vi "指数电压信号.vi"() -> ()   [LabVIEW 2020]
doc: "I. Description:\nThis example demonstrates how to output multiple Voltage Updates (Samples) to an Analog Output Channel in a software timed loop.\n\nII. Instructions for Running:\n1. Select the Physical Channel to correspond to where your signal is output on the DAQ device.\n2. Enter the Minimum and Maximum Voltage Ranges\nNote: Use the Cont Acq Multiple Samples example to verify you are generating the correct output on the DAQ device.\n3. Set the loop rate.\n4. Run theVI.\n5. Stop the VI when desired.\n\nIII. Block Diagram Steps:\n1. Create an Analog Output Voltage channel.\n2. The Array Data is a sinewave with 1000 points, generates 5 cycles, and has an amplitude of 2.\n3. Call the Start VI\n4. Write one data point from the array (modulo indexed to loop count) until the user hits the stop button or an error occurs. The loop rate is settable to 1 millisecond. \n5. Call the Clear Task VI to clear the Task.\n6. Use the popup dialog box to display an error if any. \n\nIV. I/O Connections Overview:\nMake sure your signal output terminal matches the Physical Channel I/O Control. For further connection information, refer to your hardware reference manual."
uses:
  <vilib>/Analysis/polynomials.llb/Scalar Polynomial Evaluation (DBL).vi
  GlobalVariable.vi
  <vilib>/Analysis/NI_AALPro.lvlib
panel:
  in  "定值电压输出":bool
  in  "当前输出电压":dbl format="%#.4f"
  in  "倍周期(秒)":dbl=80.0
  in  "开始":bool
  in  "输出通道选择":u16(ring) items=["电压输出一", "电压输出二", "电压输出三", "电压输出四"]
  in  "V(0)电压(V)":dbl=0.1
  in  "Stop":bool caption="stop"
  in  "Loop Time (ms)":u32=200 caption="点间步长(mS)"
  out "XY Graph":cluster{"Y":dbl[], "Y":dbl[]}[](graph) caption="指数电压输出"
  # "V(t)=V(0)exp(t/Te)"
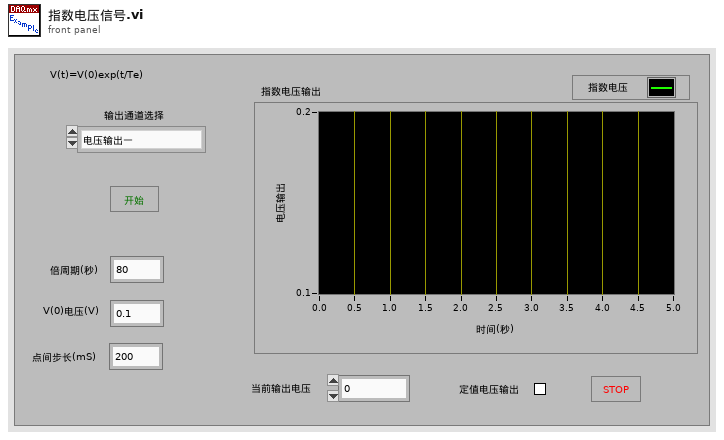
[diagram p1: front panel]
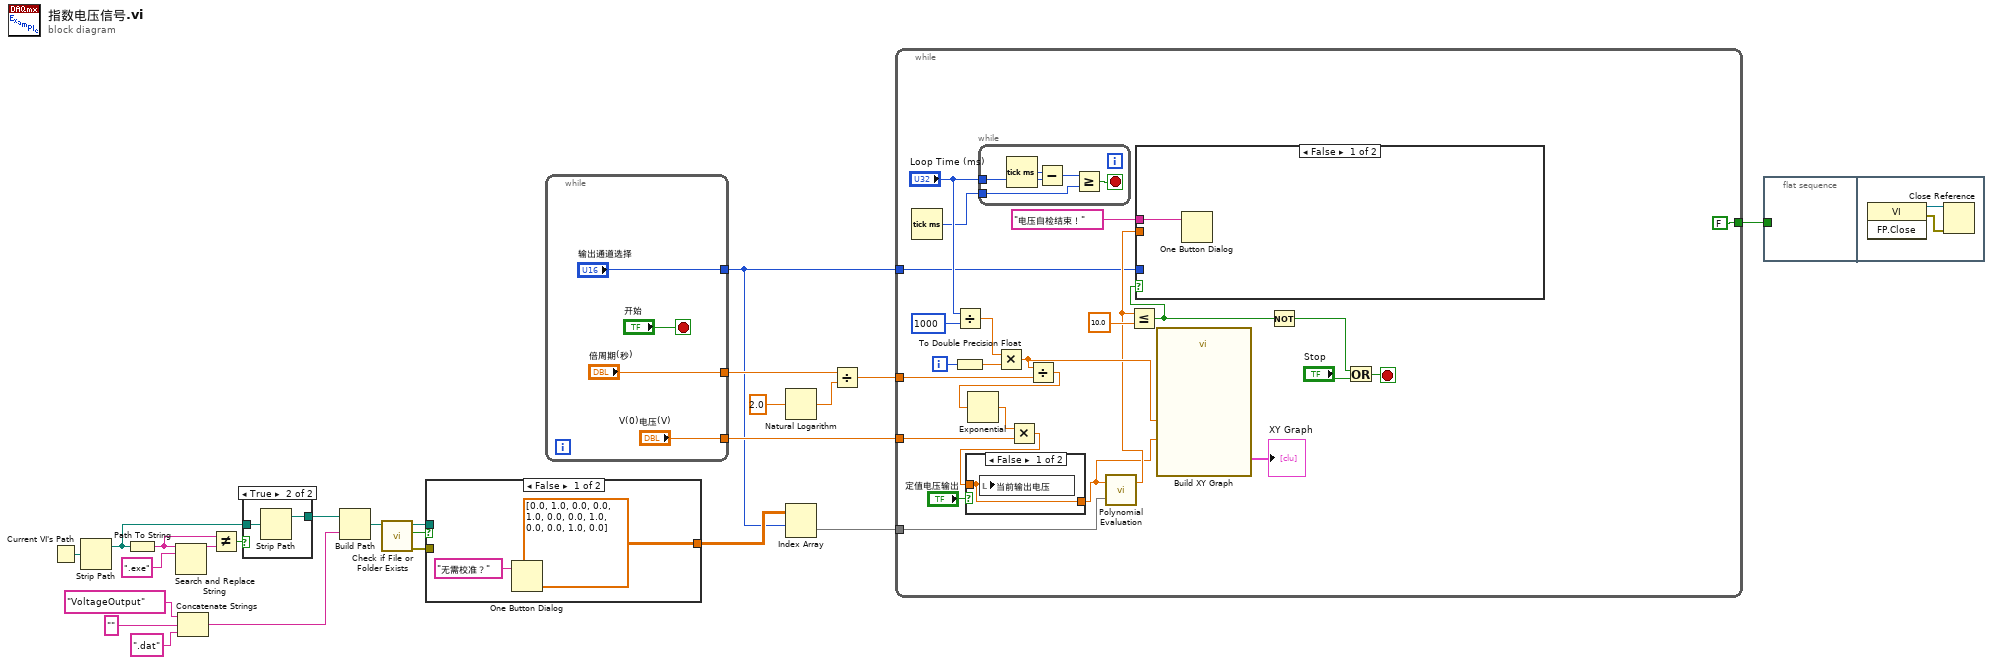
[diagram p0: block diagram]
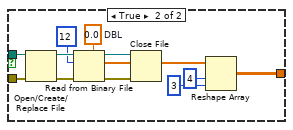
[diagram p2: hidden frame]
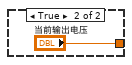
[diagram p4: hidden frame]
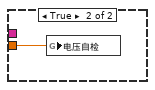
[diagram p5: hidden frame]
diagram:
  n1 = Current VI's Path() -> (path=w18:path)
  n2 = Strip Path(path=w18) -> (stripped path=w13:path)  [unwired: 1 out]
  n3 = Path To String(path=w13) -> (string=w15:string)
  n4 = Search and Replace String(input string=w15, search string=".exe" ("搜索字符串")) -> (result string=w16:string)  [unwired: 6 in, 3 out]
  n5 = Concatenate Strings("VoltageOutput", "" ("字符串"), ".dat") -> (w8:string)
  n6 = Not Equal?(x=w15, y=w16) -> (x != y?=w14:bool)
  n7 = case shown="True" w14 {
    tunnel: w13 -> [w25 w27]
    tunnel: [w25 w26] -> w12
    frame False {
    }
    frame True {
      n8 = Strip Path(path=w27) -> (stripped path=w26:path)  [unwired: 1 out]
    }
  }
  n9 = Build Path(base path=w12, name or relative path=w8) -> (appended path=w7:path)
  n10 = call <vilib>:"Check if File or Folder Exists.vi"("path"=w7) -> ("error out"=w5:errorcluster, "file or folder exists?"=w4:bool, "dup path"=w6:path)  [unwired: 8 in]
  n11 = case shown="False" w4 {
    tunnel: [dbl[][] [[0.0, 1.0, 0.0], [0.0, 1.0, 0.0], [0.0, 1.0, 0.0], [0.0, 1.0, 0.0]] w34] -> w11
    tunnel: w6 -> [_ w31]
    tunnel: w5 -> [_ w30]
    frame False {
      n12 = One Button Dialog(message="无需校准？" ("消息")) -> ()  [unwired: 1 in, 1 out]
    }
    frame True {
      w38 = 0.0  # DBL
      n13 = Open/Create/Replace File(file path (use dialog)=w31, error in=w30) -> (refnum out=w41:refnum<file>, error out=w40:errorcluster)  [unwired: 4 in, 1 out]
      n14 = Read from Binary File(5:w38, 8:w40, 10:12 ("count"), 11:w41) -> (0:w32:errorcluster, 2:w35:dbl[], 3:w33:refnum<file>)  [unwired: 2 in, 1 out]
      n15 = Close File(refnum=w33, error in=w32) -> ()  [unwired: 2 out]
      n16 = Reshape Array(w35, 4 ("维数大小"), 3 ("维数大小")) -> (w34:dbl[][])
    }
  }
  n17 = while {
    tunnel: ["倍周期(秒)"] -> w21
    tunnel: ["V(0)电压(V)"] -> w20
    tunnel: ["输出通道选择"] -> w2
    stop <- "开始" stop-if-true
  }
  n18 = Natural Logarithm(1:2.0 ("x")) -> (0:w23:dbl)
  n19 = Index Array(array=w11, index (row)=w2) -> (element=w19:dbl[])  [unwired: 1 in]
  n20 = Divide(x=w21, y=w23) -> (x/y=w24:dbl)
  n21 = while {
    tunnel: w24 -> [w66]
    tunnel: w20 -> [w64]
    tunnel: w19 -> [w55]
    tunnel: [FALSE ("非x?")] -> w3
    tunnel: w2 -> [w46]
    i -> [w68]
    stop <- w70 stop-if-true
    n22 = Tick Count (ms)() -> (millisecond timer value=w52:u32)
    n23 = Divide(x="Loop Time (ms)", y=u32 1000) -> (x/y=w61:dbl)
    n24 = To Double Precision Float(number=w68) -> (double precision float=w67:dbl)
    n25 = while {
      tunnel: "Loop Time (ms)" -> [w76]
      tunnel: w52 -> [w73]
      stop <- w74 stop-if-true
      n26 = Tick Count (ms)() -> (millisecond timer value=w77:u32)
      n27 = Subtract(x=w77, y=w76) -> (x-y=w75:u32)
      n28 = Greater Or Equal?(x=w75, y=w73) -> (x >= y?=w74:bool)
    }
    n29 = Multiply(x=w61, y=w67) -> (x*y=w59:dbl)
    n30 = Divide(x=w59, y=w66) -> (x/y=w65:dbl)
    n31 = Exponential(1:w65) -> (0:w63:dbl)
    n32 = Multiply(x=w63, y=w64) -> (x*y=w49:dbl)
    n33 = case shown="False" "定值电压输出" {
      tunnel: [w71 "当前输出电压"] -> w50
      tunnel: w49 -> [w71 _]
      frame False {
        n34 = local write "当前输出电压"(w71) -> ()
      }
      frame True {
      }
    }
    n35 = call-poly <vilib>:"Polynomial Evaluation.vi"("P(x)"=w55, "a"=w50) -> ("P(a)"=w54:dbl)  [unwired: 1 out]
    n36 = Less Or Equal?(x=w54, y=10.0) -> (x <= y?=w57:bool)
    n37 = case shown="False" w57 {
      tunnel: w54 -> [_ w79]
      tunnel: "电压自检结束！" ("消息") -> [w78 _]
      tunnel: w46 -> [_ _]
      frame False {
        n38 = One Button Dialog(message=w78) -> ()  [unwired: 1 in, 1 out]
      }
      frame True {
        n39 = global write "GlobalVariable.vi" "电压自检"(w79) -> ()
      }
    }
    n40 = call "Build XY Graph"("Y Input"=w50, "X Input"=w59) -> ("XY Graph"=→"XY Graph":cluster{"Y":dbl[], "Y":dbl[]}[])  [unwired: 3 in, 6 out]
    n41 = Not(x=w57) -> (.not. x?=w48:bool)
    n42 = Or(x=w48, y="Stop") -> (x .or. y?=w70:bool)
  }
  n43 = flat-sequence {
    tunnel: w3 -> [_]
    frame #0 {
    }
    frame #1 {
      n44 = invoke class="VI" method="FP.Close"() -> (reference out=w81:refnum<vi>, error out=w80:errorcluster)  [unwired: 3 in, 1 out]
      n45 = Close Reference(reference=w81, error in (no error)=w80) -> ()  [unwired: 1 out]
    }
  }
